vi "Find Min Max.vi"(10 "chunk size":i32, 11 "Input Array":dbl[](array[numeric])) -> (2 "Min array":dbl[](array[numeric]), 3 "Max array":dbl[](array[numeric]))   [LabVIEW 2021, in "PMIC Common.lvlib"]
doc: "Find the maximum and minimum for each chunk size from the beginning of the input array, and return arrays of maximum and minimum values."
uses:
  PMIC Common.lvlib
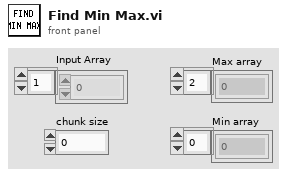
[diagram p1: front panel]
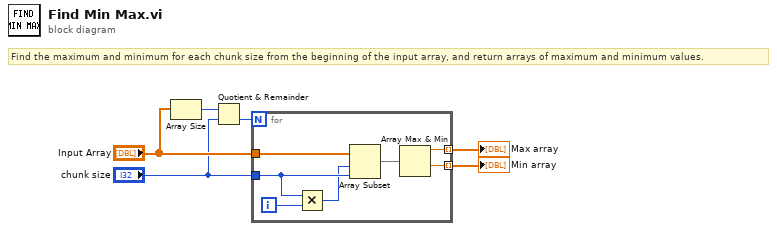
[diagram p0: block diagram]
diagram:
  # "Find the maximum and minimum for each chunk size from the beginning of the input array, and return arrays of maximum and minimum values."
  n1 = Array Size(array="Input Array") -> (size(s)=w6:i32)
  n2 = Quotient & Remainder(x=w6, y="chunk size") -> (floor(x/y)=w1:i32)  [unwired: 1 out]
  n3 = for {
    N: w1 -> [_]
    tunnel: "Input Array" -> [w13]
    tunnel: "chunk size" -> [w11]
    tunnel: [w8] -> w3 mode=indexing
    tunnel: [w7] -> w2 mode=indexing
    i -> [w12]
    n4 = Multiply(x=w11, y=w12) -> (x*y=w10:i32)
    n5 = Array Subset(array=w13, index=w10, length=w11) -> (w9:dbl[])
    n6 = Array Max & Min(array=w9) -> (max value=w8:dbl, min value=w7:dbl)  [unwired: 2 out]
  }
  "Max array" <- w3
  "Min array" <- w2
